vi "lights_create.vi"   [LabVIEW 2011]
uses:
  <vilib>/Rock Robotics/SystemInterfaces/DIO/FPGA_DIORelayChannel.ctl
  <vilib>/Rock Robotics/SystemInterfaces/Typedef/FPGA_TypedefDigitalModule.ctl
  <vilib>/Rock Robotics/WPI/Relay/WPI_RelayDirection.ctl
types:
  T1 = typedef "WPI_RelayDirection.ctl" = enum16{"Both directions", "Forward only", "Reverse only"}
  T2 = typedef "FPGA_DIORelayChannel.ctl" = enum8{"Relay 1", "Relay 2", "Relay 3", "Relay 4", "Relay 5", "Relay 6", "Relay 7", "Relay 8", "Invalid"}
  T3 = typedef "FPGA_TypedefDigitalModule.ctl" = enum16{"Digital Module 1", "Digital Module 2"}
  T4 = typedef "WPI_RelayDevRef.ctl" = cluster{"DevStatus":errorcluster, "Relay Channel":T2, "Digital Module":T3, "Relay Direction":T1}
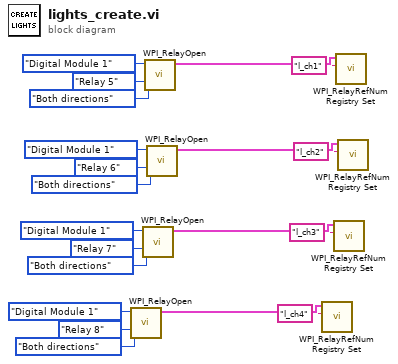
[diagram p0: block diagram]
diagram:
  n1 = call <vilib>:"WPI_RelayOpen.vi"("Relay Direction"=WPI_RelayDirection."Both directions", "Relay Channel"=FPGA_DIORelayChannel."Relay 8", "Digital Module (Module 1)"=FPGA_TypedefDigitalModule."Digital Module 1") -> ("RelayDevRef"=w2:T4)  [unwired: 7 in, 1 out]
  n2 = call <vilib>:"WPI_RelayOpen.vi"("Relay Direction"=WPI_RelayDirection."Both directions", "Relay Channel"=FPGA_DIORelayChannel."Relay 7", "Digital Module (Module 1)"=FPGA_TypedefDigitalModule."Digital Module 1") -> ("RelayDevRef"=w7:T4)  [unwired: 7 in, 1 out]
  n3 = call <vilib>:"WPI_RelayOpen.vi"("Relay Direction"=WPI_RelayDirection."Both directions", "Relay Channel"=FPGA_DIORelayChannel."Relay 5", "Digital Module (Module 1)"=FPGA_TypedefDigitalModule."Digital Module 1") -> ("RelayDevRef"=w17:T4)  [unwired: 7 in, 1 out]
  n4 = call <vilib>:"WPI_RelayOpen.vi"("Relay Direction"=WPI_RelayDirection."Both directions", "Relay Channel"=FPGA_DIORelayChannel."Relay 6", "Digital Module (Module 1)"=FPGA_TypedefDigitalModule."Digital Module 1") -> ("RelayDevRef"=w12:T4)  [unwired: 7 in, 1 out]
  n5 = call <vilib>:"WPI_RelayRefNum Registry Set.vi"("refnum name"="l_ch4", "RelayDevRef"=w2) -> ()  [unwired: 8 in, 2 out]
  n6 = call <vilib>:"WPI_RelayRefNum Registry Set.vi"("refnum name"="l_ch3", "RelayDevRef"=w7) -> ()  [unwired: 8 in, 2 out]
  n7 = call <vilib>:"WPI_RelayRefNum Registry Set.vi"("refnum name"="l_ch1", "RelayDevRef"=w17) -> ()  [unwired: 8 in, 2 out]
  n8 = call <vilib>:"WPI_RelayRefNum Registry Set.vi"("refnum name"="l_ch2", "RelayDevRef"=w12) -> ()  [unwired: 8 in, 2 out]
